vi "IMAQ-Cluster2Device.vi"(0 "Image Device IN":cluster{"Image":T1, "errorImage":errorcluster}) -> (1 "errorImage OUT":errorcluster, 2 "Image OUT":T1)   [LabVIEW 2010]
uses:
  <vilib>/vision/Image Controls.llb/IMAQ Image.ctl
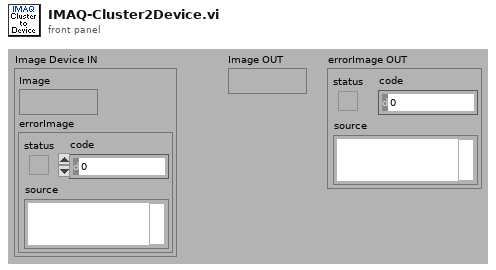
[diagram p1: front panel]
types:
  T1 = typedef "IMAQ Image.ctl" = refnum<image>
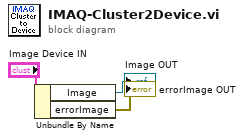
[diagram p0: block diagram]
diagram:
  n1 = Unbundle By Name("Image Device IN") -> ("Image"=→"Image OUT":T1, "errorImage"=→"errorImage OUT":errorcluster)
